vi "Insert Diagram Into Subpanel.vi"(4 "Subpanel":refnum<vi>, 5 "Method Name":string, 6 "Tag":string, 7 "Class":refnum<vi>, 8 "error in (no error)":errorcluster, 9 "Bounds in":T1, 10 "Origin in":T2, 11 "Old VI":refnum<vi>) -> (0 "error out":errorcluster, 1 "Bounds out":T1, 2 "Origin out":T2, 3 "New VI":refnum<vi>)   [LabVIEW 2020, in "Choose Implementation Dialog.lvlib"]
uses:
  Choose Implementation Dialog.lvlib
  Open Window Error Message.vi
  <vilib>/Utility/miscctls.llb/LVRectTypeDef.ctl
  <vilib>/Utility/miscctls.llb/LVPointTypeDef.ctl
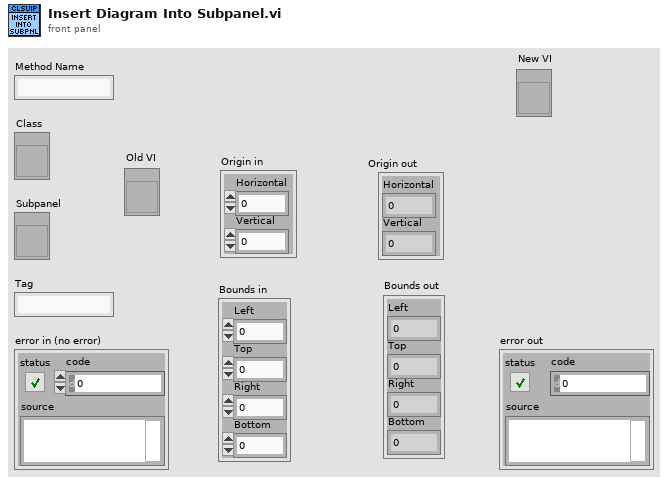
[diagram p1: front panel]
types:
  T1 = typedef "LVRectTypeDef.ctl" = cluster{"Left":i16, "Top":i16, "Right":i16, "Bottom":i16}
  T2 = typedef "LVPointTypeDef.ctl" = cluster{"Horizontal":i16, "Vertical":i16}
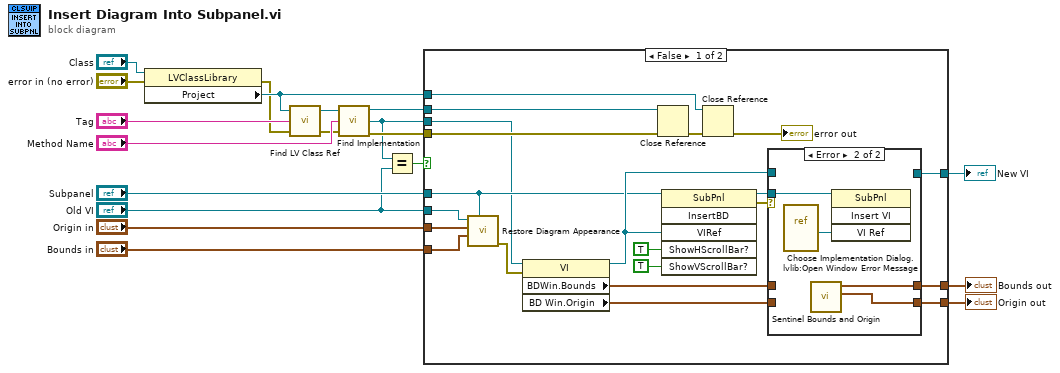
[diagram p0: block diagram]
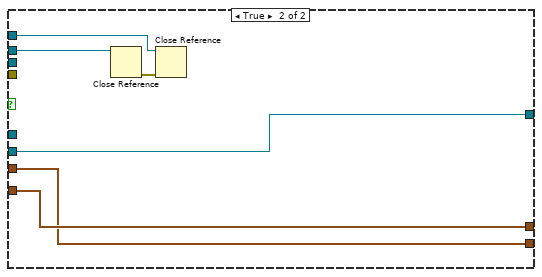
[diagram p3: hidden frame]
diagram:
  n1 = property class="LVClassLibrary"(reference="Class", error in="error in (no error)") -> (error out=w13:errorcluster, "Project"=w19:refnum<vi>)  [unwired: 1 out]
  n2 = call "Find LV Class Ref.vi"("error in (no error)"=w13, "Item ID"="Tag", "Expected Project"=w19) -> ("error out"=w11:errorcluster, "LVClassLibrary Refnum"=w10:refnum<vi>)
  n3 = call "Find Implementation.vi"("error in"=w11, "Method Name"="Method Name", "Class in"=w10) -> ("error out"=w18:errorcluster, "VI"=w3:refnum<vi>, "Class out"=w17:refnum<vi>)
  n4 = Equal?(x=w3, y="Old VI") -> (x = y?=w1:bool)
  n5 = case shown="False" w1 {
    tunnel: w19 -> [w37 w48]
    tunnel: w18 -> [w35 _]
    tunnel: w17 -> [w34 w49]
    tunnel: [w31 w53] -> w9
    tunnel: [w30 w52] -> w8
    tunnel: "Origin in" -> [w27 w52]
    tunnel: "Bounds in" -> [w26 w53]
    tunnel: [w24 w51] -> w5
    tunnel: "Subpanel" -> [w22 _]
    tunnel: w3 -> [w21 _]
    tunnel: "Old VI" -> [w20 w51]
    frame False {
      n6 = call "Restore Diagram Appearance.vi"("Subpanel"=w22, "Bounds"=w26, "Origin"=w27, "Inserted VI"=w20) -> ("error out"=w23:errorcluster)  [unwired: 7 in]
      n7 = property class="VI"(reference=w21, error in=w23) -> (reference out=w25:refnum<vi>, "BDWin.Bounds"=w29:T1, "BD Win.Origin"=w28:T2)  [unwired: 1 out]
      n8 = Close Reference(reference=w34, error in (no error)=w35) -> (error out=w36:errorcluster)
      n9 = invoke on="Invoke Node" class="SubPnl" method="InsertBD"(reference=w22, "VIRef"=w25, "ShowHScrollBar?"=TRUE ("ShowHScrollBar"), "ShowVScrollBar?"=TRUE ("ShowVScrollBar")) -> (reference out=w32:refnum<vi>, error out=w33:errorcluster)  [unwired: 2 in, 4 out]
      n10 = Close Reference(reference=w37, error in (no error)=w36) -> (error out=→"error out":errorcluster)
      n11 = case shown="Error" w33 {
        tunnel: w32 -> [_ w47]
        tunnel: [w43 w45] -> w31
        tunnel: [w42 w44] -> w30
        tunnel: w29 -> [w43 _]
        tunnel: w28 -> [w42 _]
        tunnel: w25 -> [w41 _]
        tunnel: [w41 _] -> w24
        frame No Error {
        }
        frame Error {
          n12 = vi-ref "Choose Implementation Dialog.lvlib:Open Window Error Message.vi"() -> (w46:refnum<vi>)
          n13 = call "Sentinel Bounds and Origin.vi"() -> ("Sentinel Origin"=w44:T2, "Sentinel Bounds"=w45:T1)  [unwired: 10 in]
          n14 = invoke on="Invoke Node" class="SubPnl" method="Insert VI"(reference=w47, "VI Ref"=w46) -> ()  [unwired: 2 in, 4 out]
        }
      }
    }
    frame True {
      n15 = Close Reference(reference=w49) -> (error out=w50:errorcluster)  [unwired: 1 in]
      n16 = Close Reference(reference=w48, error in (no error)=w50) -> ()  [unwired: 1 out]
    }
  }
  "Origin out" <- w8
  "Bounds out" <- w9
  "New VI" <- w5
